vi "Data Plotter Dots and Dash.vi"() -> ()   [LabVIEW 2019]
uses:
  <vilib>/Utility/file.llb/Read Delimited Spreadsheet (string).vi
  <vilib>/Analysis/NI_AALBase.lvlib
panel:
  out "Histogram Graph":T1(graph)
  in  "intervals":i32=10
  in  "String":string
  out "Difference":dbl[](array[numeric])
  in  "transpose? (F)":bool
  out "Data":string[][](array[string])
  in  "delimiter (\\t)":string="\t"
  in  "file path (dialog if empty)":path
  # "#!/usr/bin/env pybricks-micropython\n\n#VSCODE main.py\n\nfrom pybricks import ev3brick as brick\nfrom pybricks.ev3devices import (Motor, TouchSensor, ColorSensor,\n                                 InfraredSensor, UltrasonicSensor, GyroSensor)\nfrom pybricks.parameters import (Port, Stop, Direction, Button, Color,\n                                 SoundFile, ImageFile, Align)\nfrom pybricks.tools import print, wait, StopWatch\nfrom pybricks.robotics import DriveBase\nimport utime\nbrick.display.text(\"milan\")\nutime.sleep(1)\ndots=[None] *10\ndashes=[None] *10\nt=TouchSensor(Port.S1)\ndot_counter=0\ndash_counter=0\nhowmany=10\n\nf = open('data.csv', 'w')           #opens the file in write mode\n\nbrick.display.text(\"Hold down for DOTS\")\nf.write(\"Dots ,\")\nwhile True:  \n    while(t.pressed()==False):\n        print(\"\") \n    a=utime.ticks_ms()\n    while (t.pressed()):\n        print(\"\")\n    b=utime.ticks_ms()\n    brick.display.text(\"Entry \"+str(dot_counter+1)+\" \"+str(b-a)+\" ms\")\n    dots[dot_counter]=b-a\n    f.write(str(b-a)+\",\")\n    dot_counter+=1\n    if(dot_counter==howmany):\n        break\n\nf.write(\"\\nDash ,\")\nbrick.display.text(\"Hold down for DASHES\")\nwhile True:\n    while(t.pressed()==False):\n        print(\"\")\n    a=utime.ticks_ms()\n    while (t.pressed()):\n        print(\"\")\n    b=utime.ticks_ms()\n    brick.display.text(\"Entry \"+str(dash_counter+1)+\" \"+str(b-a)+\" ms\")\n    dashes[dash_counter]=b-a\n    f.write(str(b-a)+\",\")\n    dash_counter+=1\n    if(dash_counter==howmany):\n        break\nf.close()"
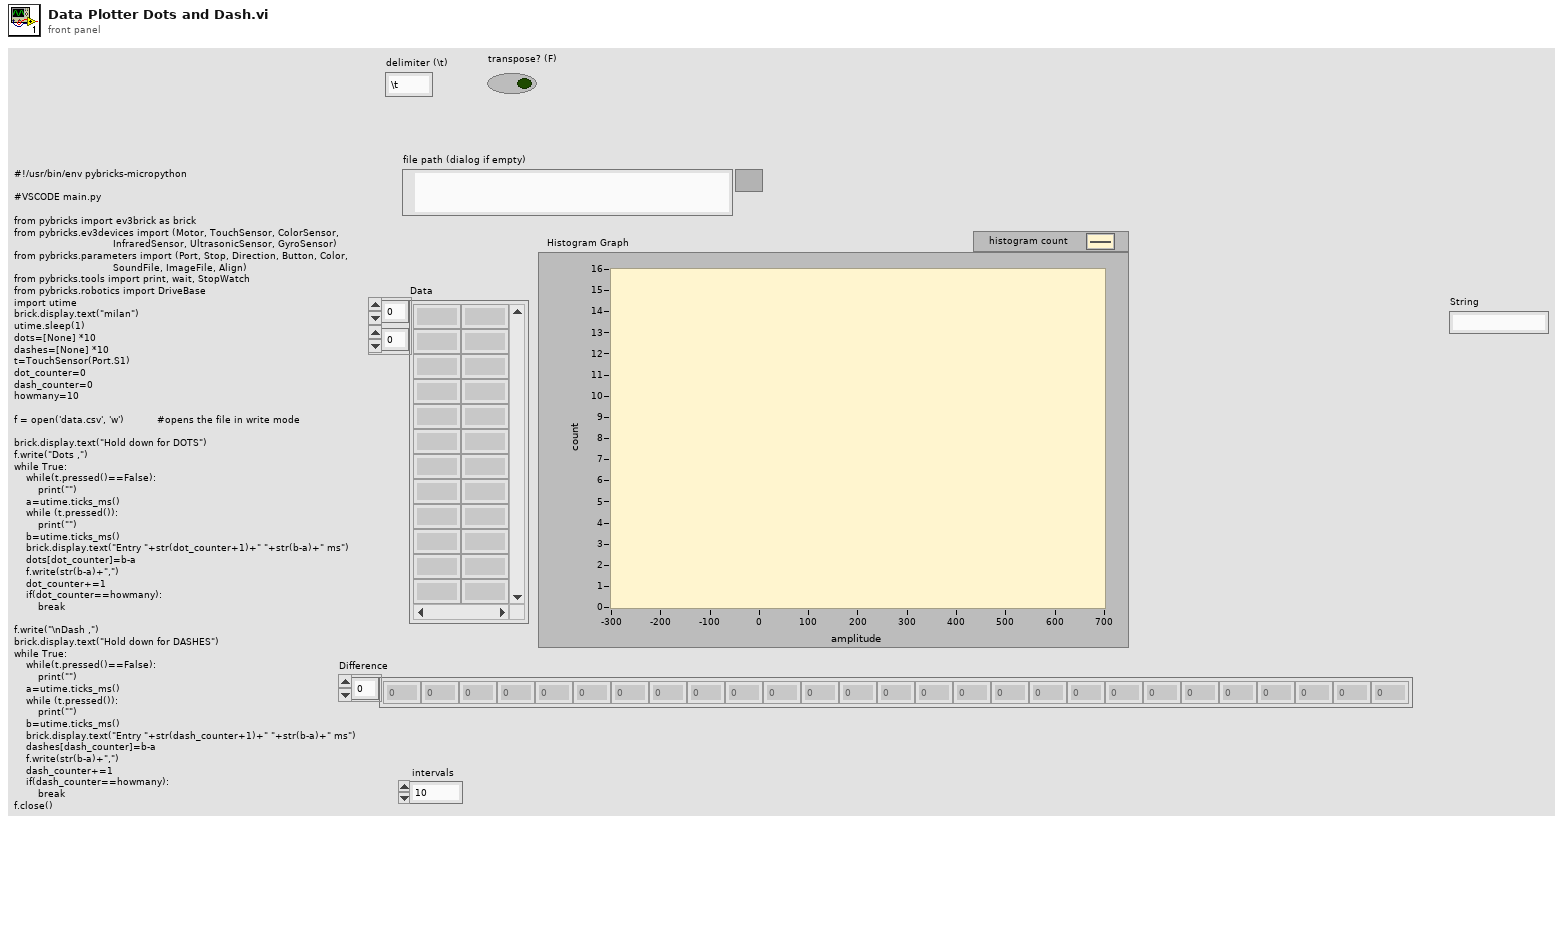
[diagram p1: front panel]
types:
  T1 = cluster{"X Values":dbl[], "Histogram: h(x)":i32[]}
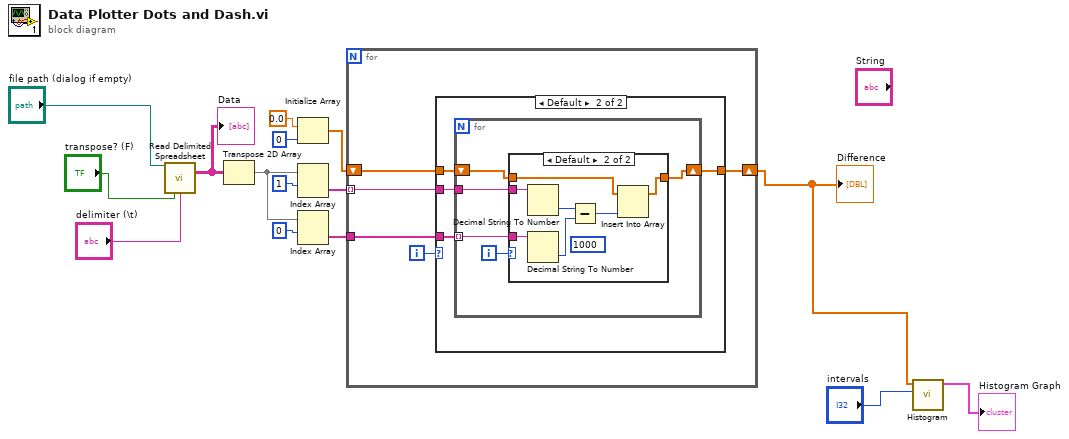
[diagram p0: block diagram]
diagram:
  n1 = call-poly <vilib>:"Read Delimited Spreadsheet.vi"("file path (dialog if empty)"="file path (dialog if empty)", "transpose? (F)"="transpose? (F)", "delimiter (\\t)"="delimiter (\\t)") -> ("all rows"=w11:string[][])  [unwired: 7 in, 5 out]
  "Data" <- w11
  n2 = Transpose 2D Array(2D array=w11) -> (transposed array=w10:string[][])
  n3 = Initialize Array(0.0 ("element"), 0 ("dimension size")) -> (w4:dbl[])
  n4 = Index Array(array=w10, index (row)=1) -> (element=w7:string[])  [unwired: 1 in]
  n5 = Index Array(array=w10, index (row)=0) -> (element=w8:string[])  [unwired: 1 in]
  n6 = for {
    tunnel: w7 -> [w20] mode=indexing
    tunnel: w8 -> [w19]
    shift-right: [w17] -> w1
    shift-left: w4 -> [w18]
    i -> [w16]
    n7 = case shown="Default" w16 {
      tunnel: w20 -> [_ w25]
      tunnel: w19 -> [_ w24]
      tunnel: w18 -> [w21 w23]
      tunnel: [w21 w22] -> w17
      frame 0 {
      }
      frame Default {
        n8 = for {
          tunnel: w25 -> [w27]
          tunnel: w24 -> [w28] mode=indexing
          shift-right: [w26] -> w22
          shift-left: w23 -> [w29]
          i -> [w30]
          n9 = case shown="Default" w30 {
            tunnel: w29 -> [w31 w35]
            tunnel: w28 -> [_ w34]
            tunnel: w27 -> [_ w33]
            tunnel: [w31 w32] -> w26
            frame 0 {
            }
            frame Default {
              (unwired) u32 1000 ("milliseconds to wait")
              n10 = Decimal String To Number(string=w33) -> (number=w36:i32)  [unwired: 2 in, 1 out]
              n11 = Decimal String To Number(string=w34) -> (number=w37:i32)  [unwired: 2 in, 1 out]
              n12 = Subtract(x=w36, y=w37) -> (x-y=w38:i32)
              n13 = Insert Into Array(array=w35, new element=w38) -> (w32:dbl[])  [unwired: 1 in]
            }
          }
        }
      }
    }
  }
  "Difference" <- w1
  n14 = call <vilib>:"Histogram.vi"("intervals"="intervals", "X"=w1) -> ("Histogram Graph"=→"Histogram Graph":T1)  [unwired: 6 in, 3 out]
